vi "Destroy Command FIFO.vi"(8 "error in (no error)":errorcluster, 11 "Thread in":refnum<class "Thread.lvclass">) -> (0 "error out":errorcluster, 3 "Thread out":refnum<class "Thread.lvclass">)   [LabVIEW 2021, in "DSF Core.lvlib" / "Thread.lvclass"]
uses:
  Thread.lvclass
  Thread.lvclass/Thread.ctl
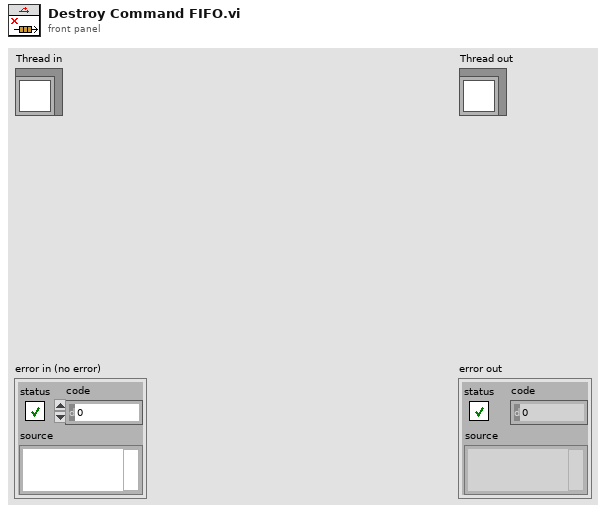
[diagram p1: front panel]
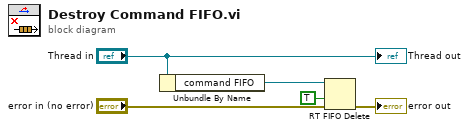
[diagram p0: block diagram]
diagram:
  n1 = Unbundle By Name("Thread in") -> ("command FIFO"=w2:refnum<k33>)
  n2 = RT FIFO Delete(0:w2, 2:TRUE ("force destroy? (F)"), 3:"error in (no error)") -> (11:→"error out":errorcluster)
  "Thread out" <- "Thread in"
